vi "Main.vi"() -> ()   [LabVIEW 2023]
doc: "This template is for the Queued Message Handler design pattern.\n\nThe Event Handling Loop generates messages based on user interface actions.\n\nThe Message Handling Loop processes messages generated by the Event Handling Loop, or by other messages. The messages are string values, so new messages can be added easily to the Message Cases case structure in the Message Handling Loop. Each message cluster can also provide an optional value for Message Data, which is a variant that can be converted to whatever message-specific data is required."
uses:
  Drivers/Resideo Gas Valve/Type Definitions/Temperature Control.ctl
  controls/UI Data.ctl
  Drivers/Resideo Gas Valve/Type Definitions/Vesta Info.ctl
  controls/Timer Application Cluster.ctl
  controls/Burner Duty Cycle.ctl
  Hybrid Water Heater/Type Definitions/HEWH MW100 Data Cluster.ctl
  Hybrid Water Heater/Custom Instrument Control/MW100/Type Definitions/HEWH Module 4 Relay Status.ctl
  support/Message Queue/Enqueue Message (Single).vi
  <vilib>/Utility/error.llb/Error Cluster From Error Code.vi
  <vilib>/ErrorRing/Error Ring.xnode
  support/Message Queue/Message Queue.lvlib
  support/User Event - Stop/User Event - Stop.lvlib
panel:
  in  "Disable T2 Control":bool
  in  "Differential Top":dbl=12.0 format="%#_13g"
  in  "Save Rate (ms)":i32=1000
  in  "MW100 Com Port":refnum<visa-resource-name>
  in  "Disable Cycling":bool=TRUE
  in  "Update Vesta Temperature":bool
  in  "VestaTemperature":T1={"Water Heater Temp (°F)"=125, "Differential  (°F)"=25.0} {"Water Heater Temp (°F)" min=32 max=203}
  in  "Burner OFF Time (Seconds)":dbl=60.0
  in  "Burner ON Time (Seconds)":dbl=60.0
  in  "Update Duty Cycle":bool
  out "Data Cluster Output":T2={"Vesta Data Output"={"Temp_W_Raw_U"=0, "Temp_W_Raw_L"=0, "Temperature Water (F)"=0.0, "Temperature Water Compensated (F)"=0.0, "Temperature Ambient (F)"=0.0, "Setpoint Location (F)"=0.0, "Heat Request"="", "Fault Ram"="", "PWM DCDC Value"=0, "Pilot Voltage (mV)"=0.0, "Setpoint Actual (F)"=0.0, "Differential Actual (F)"=0.0, "Setpoint User (F)"=0.0, "Differential User (F)"=0.0, "Termperature FIltered -TCO (F)"=0.0, "Temp_C_Raw_1 - Sensor Voltage"="", "Temp_C_Raw_2 - Sensor Voltage"="", "Chamber Sensor Temperature (F)"=0.0, "LDO Base Temperature (F)"=0.0, "LDO Timer (sec)"=0, "Disabled (0)"=FALSE, "Warming (1)"=FALSE, "Heating (2)"=FALSE, "Cooling Data Write (3)"=FALSE, "Cooling (4)"=FALSE, "Data Read (5)"=FALSE, "N/A"=FALSE, "Temperature Trip (7)"=FALSE, "Burner"=FALSE}, "VestaTemperature"={"Water Heater Temp (°F)"=135, "Differential  (°F)"=10.0}, "Timer Application Data"={"Duty Cycle"={"Burner ON Time (Seconds)"=60.0, "Burner OFF Time (Seconds)"=60.0, "Main Burner Flag"=FALSE, "Burner Power Mode"=0}}, "Data Array"=[], "MW Output"={"TC1-Channel 021"=0.0, "TC2-Channel 022"=0.0, "TC3-Channel 023"=0.0, "TC4-Channel 024"=0.0, "TC5-Channel 025"=0.0, "TC6-Channel 026"=0.0, "TC7-Channel 017"=0.0, "TC8-Channel 028"=0.0, "TC9-Channel 029"=0.0, "TC10-Channel 030"=0.0, "TC Tree Average"=0.0, "TC DWN- Channel 027"=0.0, "RTDin-Channel 031"=0.0, "RTDout-Channel 032"=0.0, "RTDamb-Channel 033"=0.0, "PSI1-Channel 011"=0.0, "PSI2-Channel 012"=0.0, "PSI3-Channel 013"=0.0, "PSI4-Channel 014"=0.0, "UE State-Channel 015"=0.0, "LE State-Channel 016"=0.0, "Module 4 Relay Status Output"={"INTELLIFAUCET TEMP(T)/FLOW(F) (CH 041)"=FALSE, "INTELLIFAUCET READY (CH 042)"=FALSE, "INTELLIFAUCET START (CH 043)"=FALSE, "INTELLIFAUCET STOP (CH 044)"=FALSE, "MAIN POWER RELAY (CH 047)"=FALSE, "NOT USED (CH 045)"=FALSE, "NOT USED (CH 046)"=FALSE, "PURGE VALVE RELAY (CH 048)"=FALSE, "OUTLET VALVE RELAY (CH 049)"=FALSE, "INLET VALVE RELAY (CH 050)"=FALSE, "Intellifaucet (% Open)"=0.0, "Proportioning Valve (%Open)"=0.0, "Intellifaucet Temp Setpoint (F)"=0.0}}} {"VestaTemperature"."Water Heater Temp (°F)" min=32 max=203}
  in  "Vesta Com Port":refnum<visa-resource-name>
  out "Debug":string[](array[string])
  in  "Debug":bool
  in  "Save Data":bool
  in  "Exit":bool
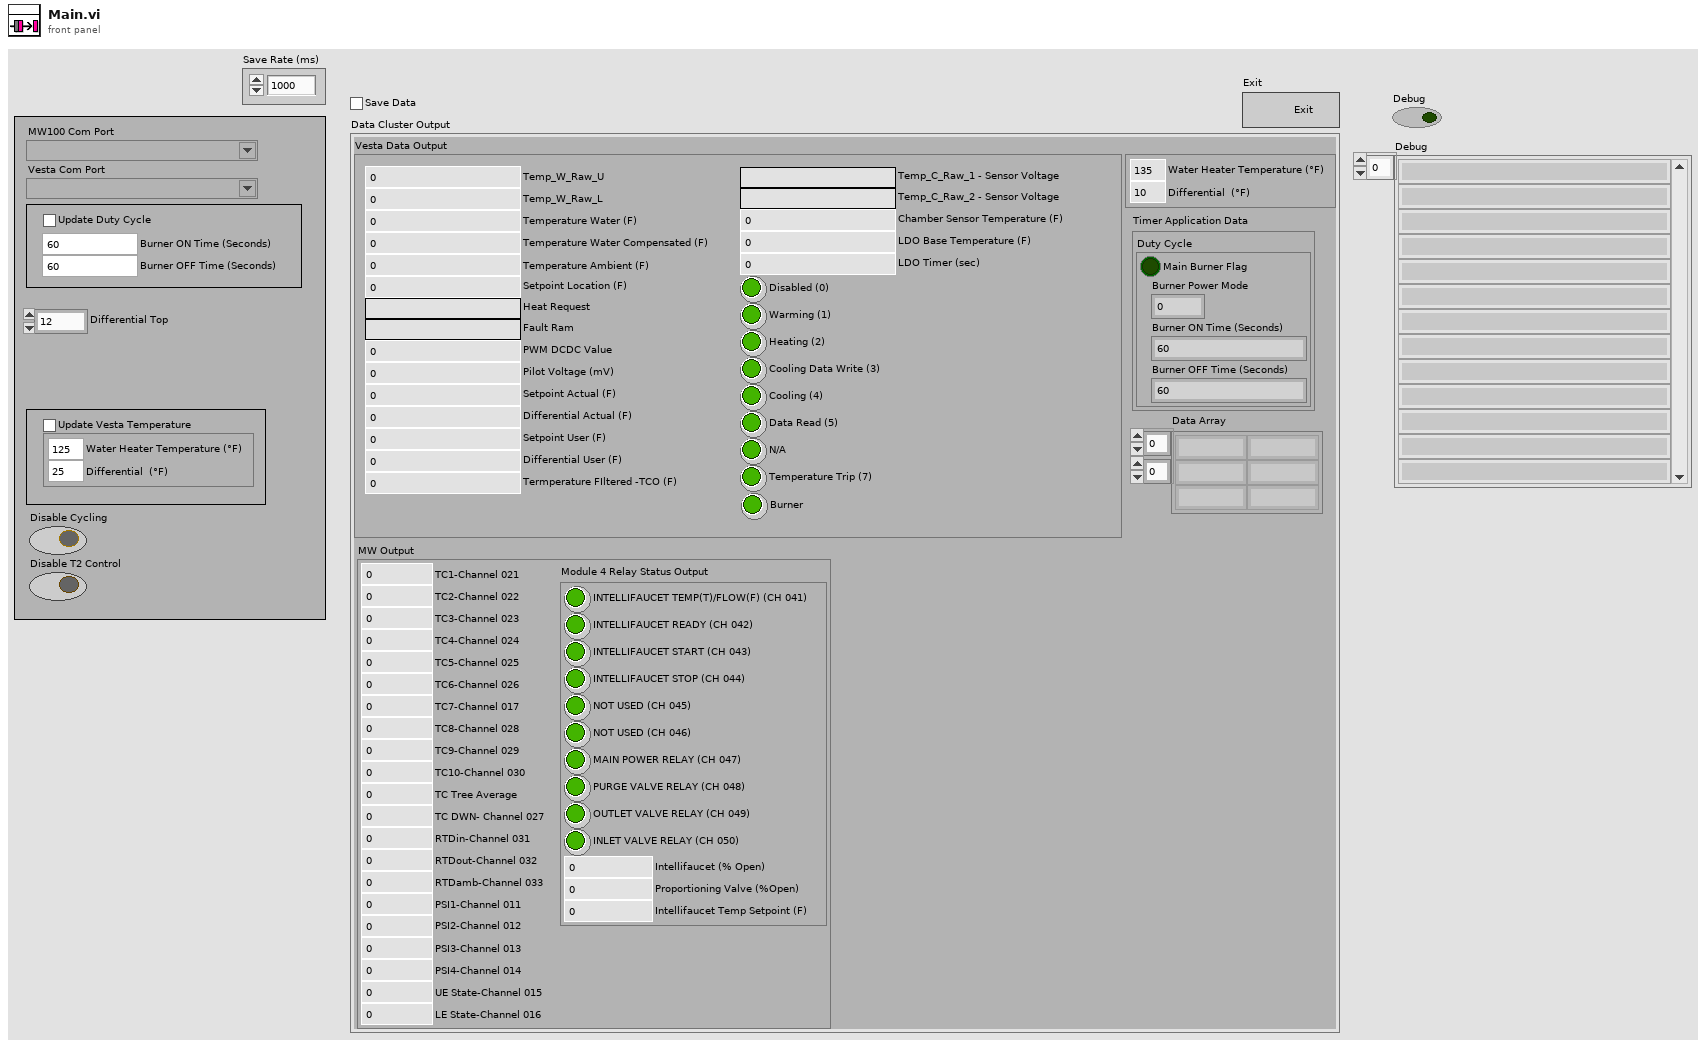
[diagram p1: front panel]
types:
  T1 = typedef "Temperature Control.ctl" = cluster{"Water Heater Temp (°F)":u16, "Differential  (°F)":dbl}
  T2 = typedef "UI Data.ctl" = cluster{"Vesta Data Output":T3, "VestaTemperature":T1, "Timer Application Data":T4, "Data Array":string[][], "MW Output":T6}
  T3 = typedef "Vesta Info.ctl" = cluster{"Temp_W_Raw_U":u16, "Temp_W_Raw_L":u16, "Temperature Water (F)":dbl, "Temperature Water Compensated (F)":dbl, "Temperature Ambient (F)":dbl, "Setpoint Location (F)":dbl, "Heat Request":string, "Fault Ram":string, "PWM DCDC Value":u16, "Pilot Voltage (mV)":dbl, "Setpoint Actual (F)":dbl, "Differential Actual (F)":dbl, "Setpoint User (F)":dbl, "Differential User (F)":dbl, "Termperature FIltered -TCO (F)":dbl, "Temp_C_Raw_1 - Sensor Voltage":string, "Temp_C_Raw_2 - Sensor Voltage":string, "Chamber Sensor Temperature (F)":dbl, "LDO Base Temperature (F)":dbl, "LDO Timer (sec)":i16, "Disabled (0)":bool, "Warming (1)":bool, "Heating (2)":bool, "Cooling Data Write (3)":bool, "Cooling (4)":bool, "Data Read (5)":bool, "N/A":bool, "Temperature Trip (7)":bool, "Burner":bool}
  T4 = typedef "Timer Application Cluster.ctl" = cluster{"Duty Cycle":T5}
  T5 = typedef "Burner Duty Cycle.ctl" = cluster{"Burner ON Time (Seconds)":dbl, "Burner OFF Time (Seconds)":dbl, "Main Burner Flag":bool, "Burner Power Mode":u8}
  T6 = typedef "HEWH MW100 Data Cluster.ctl" = cluster{"TC1-Channel 021":dbl, "TC2-Channel 022":dbl, "TC3-Channel 023":dbl, "TC4-Channel 024":dbl, "TC5-Channel 025":dbl, "TC6-Channel 026":dbl, "TC7-Channel 017":dbl, "TC8-Channel 028":dbl, "TC9-Channel 029":dbl, "TC10-Channel 030":dbl, "TC Tree Average":dbl, "TC DWN- Channel 027":dbl, "RTDin-Channel 031":dbl, "RTDout-Channel 032":dbl, "RTDamb-Channel 033":dbl, "PSI1-Channel 011":dbl, "PSI2-Channel 012":dbl, "PSI3-Channel 013":dbl, "PSI4-Channel 014":dbl, "UE State-Channel 015":dbl, "LE State-Channel 016":dbl, "Module 4 Relay Status Output":T7}
  T7 = typedef "HEWH Module 4 Relay Status.ctl" = cluster{"INTELLIFAUCET TEMP(T)/FLOW(F) (CH 041)":bool, "INTELLIFAUCET READY (CH 042)":bool, "INTELLIFAUCET START (CH 043)":bool, "INTELLIFAUCET STOP (CH 044)":bool, "MAIN POWER RELAY (CH 047)":bool, "NOT USED (CH 045)":bool, "NOT USED (CH 046)":bool, "PURGE VALVE RELAY (CH 048)":bool, "OUTLET VALVE RELAY (CH 049)":bool, "INLET VALVE RELAY (CH 050)":bool, "Intellifaucet (% Open)":dbl, "Proportioning Valve (%Open)":dbl, "Intellifaucet Temp Setpoint (F)":dbl}
  T8 = typedef "Message Queue.lvlib/All Message Queues.ctl" = cluster{"UI":refnum<queue>, "DataSave":refnum<queue>, "Vesta":refnum<queue>, "MW100":refnum<queue>}
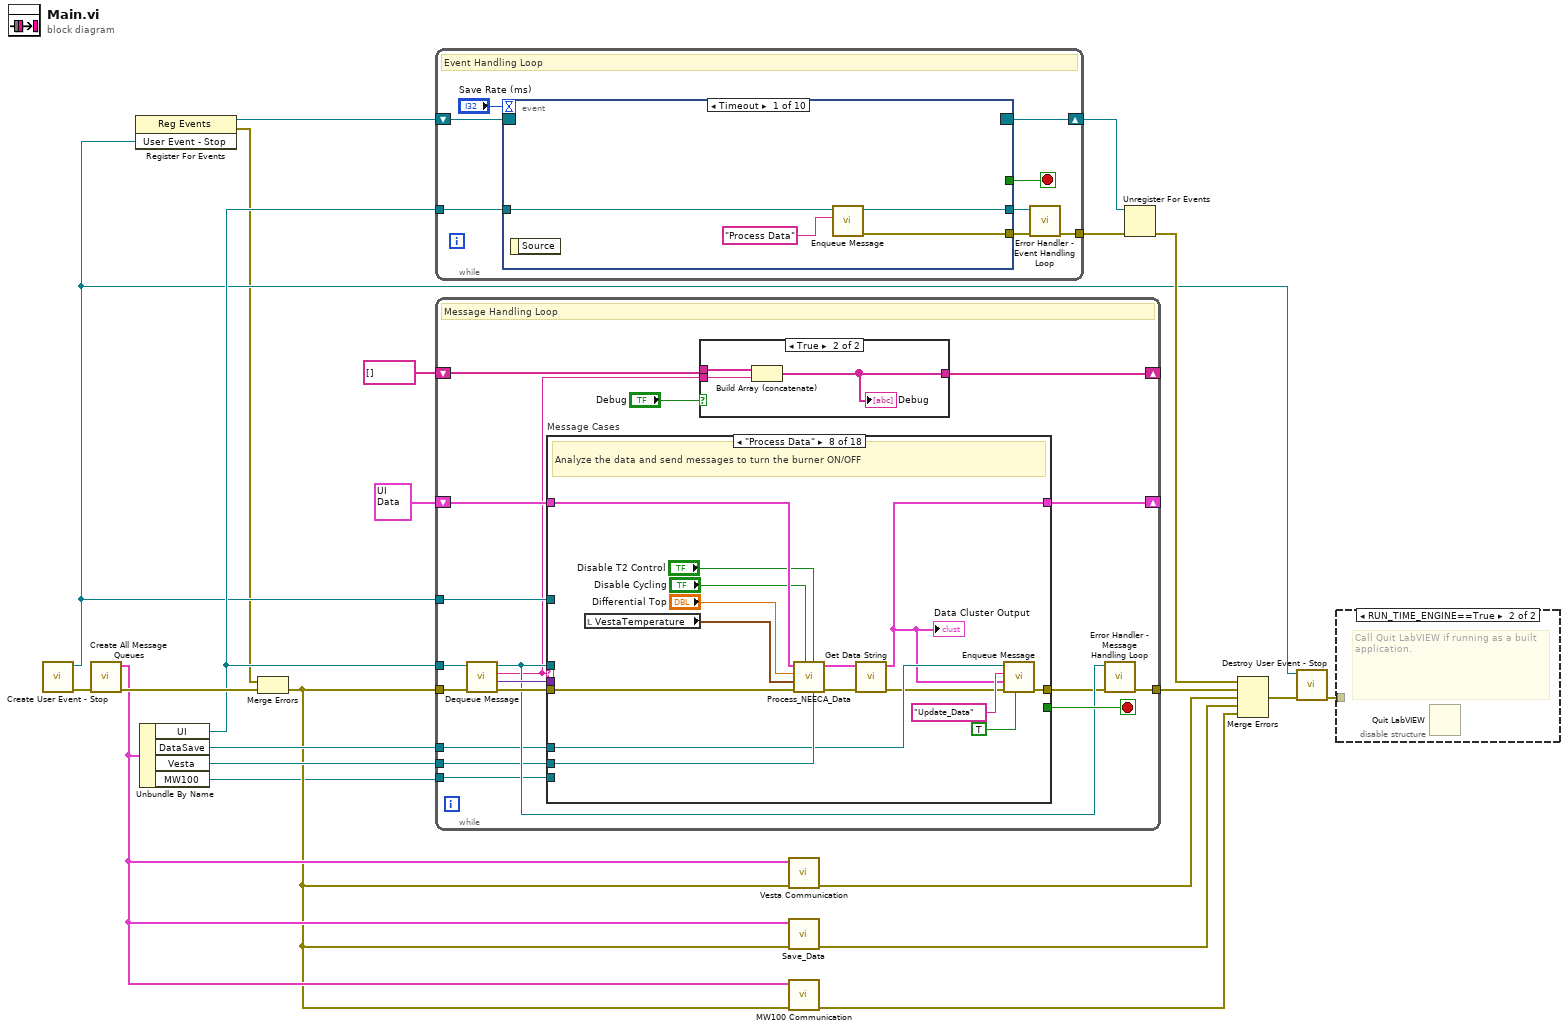
[diagram p0: block diagram]
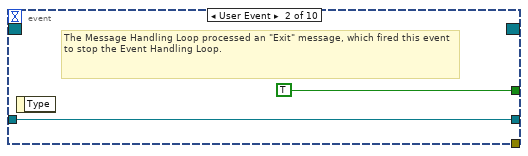
[diagram p3: hidden frame]
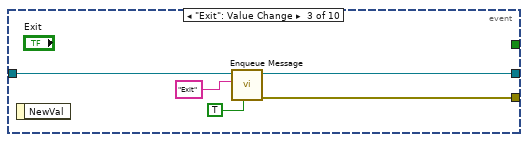
[diagram p4: hidden frame]
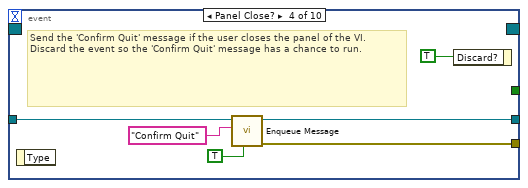
[diagram p5: hidden frame]
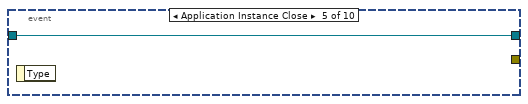
[diagram p6: hidden frame]
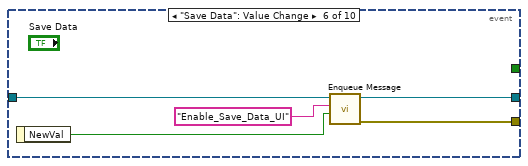
[diagram p7: hidden frame]
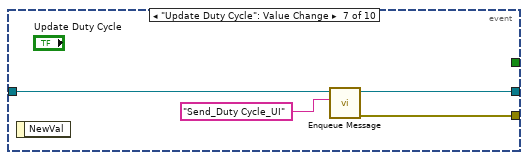
[diagram p8: hidden frame]
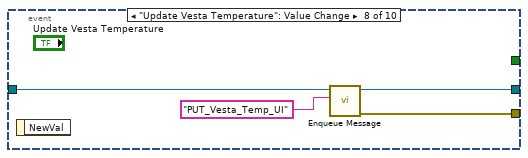
[diagram p9: hidden frame]
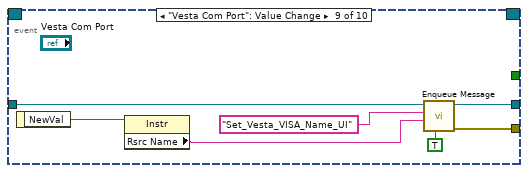
[diagram p10: hidden frame]
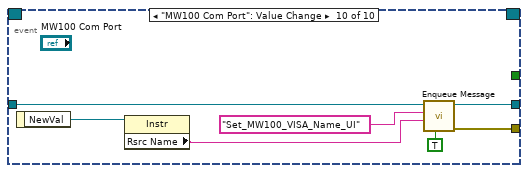
[diagram p11: hidden frame]
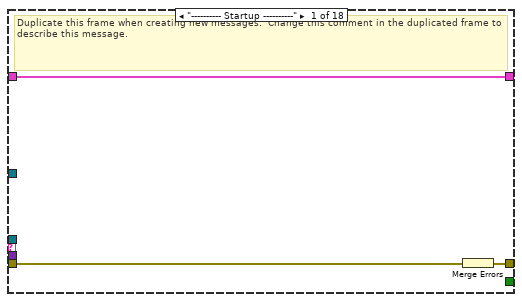
[diagram p13: hidden frame]
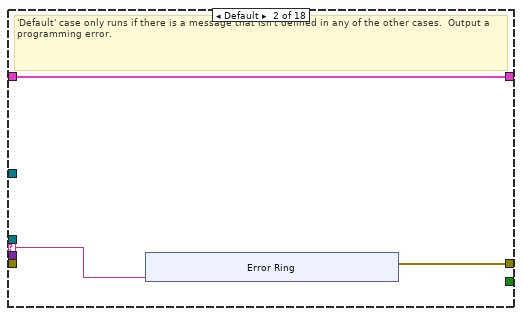
[diagram p14: hidden frame]
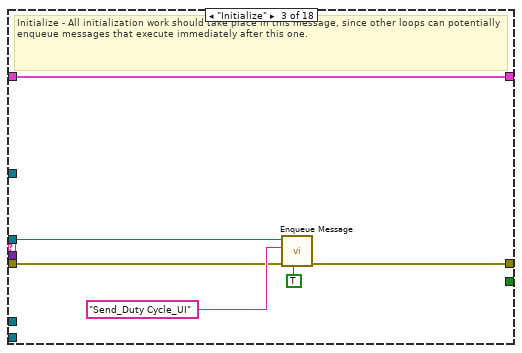
[diagram p15: hidden frame]
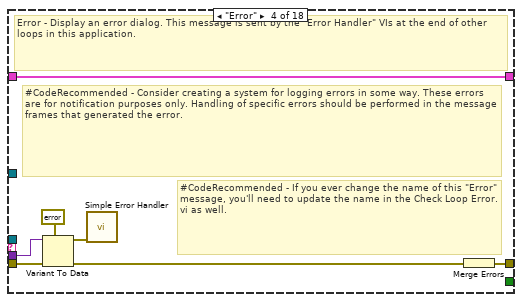
[diagram p16: hidden frame]
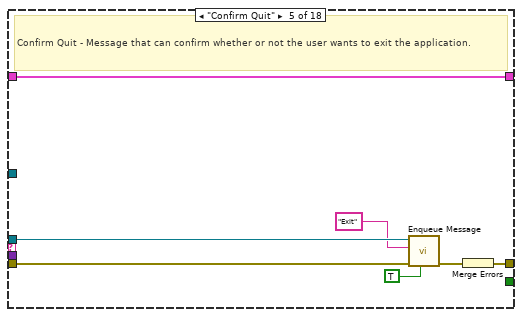
[diagram p17: hidden frame]
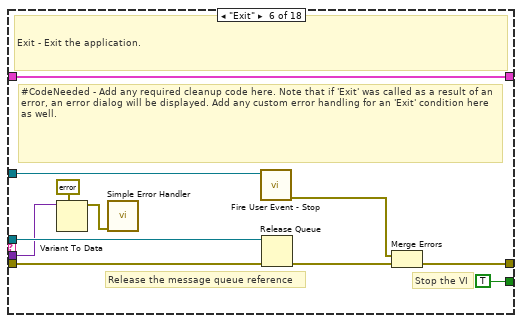
[diagram p18: hidden frame]
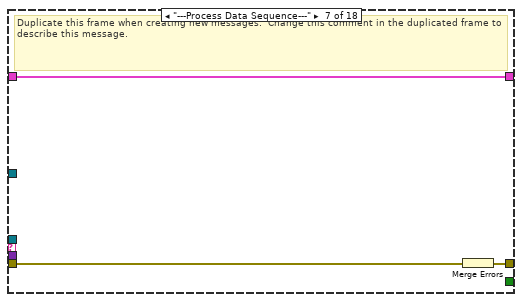
[diagram p19: hidden frame]
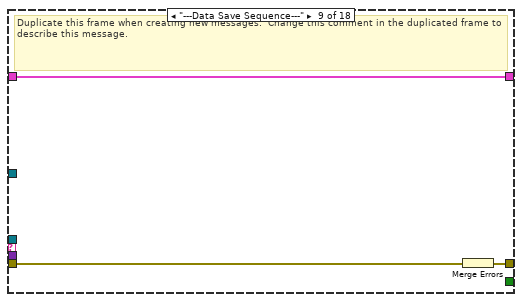
[diagram p20: hidden frame]
diagram:
  n1 = call "Create User Event - Stop.vi"() -> ("error out"=w19:errorcluster, "User Event - Stop"=w11:refnum<user-event>)  [unwired: 10 in]
  n2 = call "Create All Message Queues.vi"("error in (no error)"=w19) -> ("error out"=w22:errorcluster, "Message Queues out"=w4:T8)  [unwired: 9 in]
  n3 = register-events(w11) -> (reference out=w12:refnum<event-registration>, error out=w10:errorcluster)  [unwired: 2 in]
  n4 = Unbundle By Name(w4) -> ("UI"=w20:refnum<queue>, "DataSave"=w9:refnum<queue>, "Vesta"=w6:refnum<queue>, "MW100"=w1:refnum<queue>)
  n5 = Merge Errors(w10, w22) -> (w3:errorcluster)
  n6 = while {
    tunnel: w20 -> [w30]
    shift-right: [w28] -> w16
    shift-left: w12 -> [w29]
    tunnel: [w24] -> w13
    stop <- w26 stop-if-true
    # "Event Handling Loop"
    n7 = event shown="[0] Timeout" {
      selector: w29 -> [_ _ _ _ _ _ _ _ _ _]
      dyn-events: [_ _ _ _ _ _ _ _ _ _] -> w28
      timeout: "Save Rate (ms)" -> [_ _ _ _ _ _ _ _ _ _]
      tunnel: [_ TRUE ("Discard?") _ _ _ _ _ _ _ _] -> w26
      tunnel: w30 -> [w33 w36 w41 w46 w48 w53 w57 w61 w68 w75]
      tunnel: [w31 _ w40 w45 _ w50 w54 w58 w65 w72] -> w27
      tunnel: [w32 w36 w39 w44 w48 w52 w56 w60 w67 w74] -> w25
      event Timeout {
        n8 = event-data() -> ()  [unwired: 1 in, 1 out]
        n9 = call-poly "Enqueue Message.vi"("Message"="Process Data", "Message Queue"=w33) -> ("error out"=w31:errorcluster, "dup Message Queue"=w32:refnum<queue>)  [unwired: 8 in]
      }
      event User Event {
        # "The Message Handling Loop processed an \"Exit\" message, which fired this event to stop the Event Handling Loop."
        n10 = event-data() -> ()  [unwired: 1 in, 1 out]
      }
      event "Exit": Value Change {
        n11 = event-data() -> ()  [unwired: 1 in, 1 out]
        n12 = call-poly "Enqueue Message.vi"("Priority Message? (F)"=TRUE, "Message"="Exit", "Message Queue"=w41) -> ("error out"=w40:errorcluster, "dup Message Queue"=w39:refnum<queue>)  [unwired: 7 in]
      }
      event Panel Close? {
        # "Send the 'Confirm Quit' message if the user closes the panel of the VI. Discard the event so the 'Confirm Quit' message has a chance to run."
        n13 = event-data() -> ()  [unwired: 1 in, 1 out]
        n14 = call-poly "Enqueue Message.vi"("Priority Message? (F)"=TRUE, "Message"="Confirm Quit", "Message Queue"=w46) -> ("error out"=w45:errorcluster, "dup Message Queue"=w44:refnum<queue>)  [unwired: 7 in]
        n15 = event-data("Discard?"=TRUE) -> ()  [unwired: 1 in, 1 out]
      }
      event Application Instance Close {
        n16 = event-data() -> ()  [unwired: 1 in, 1 out]
      }
      event "Save Data": Value Change {
        n17 = event-data() -> ("NewVal"=w49:bool)  [unwired: 1 in]
        n18 = call-poly "Enqueue Message.vi"("Message Data"=w49, "Message"="Enable_Save_Data_UI", "Message Queue"=w53) -> ("error out"=w50:errorcluster, "dup Message Queue"=w52:refnum<queue>)  [unwired: 7 in]
      }
      event "Update Duty Cycle": Value Change {
        n19 = event-data() -> ()  [unwired: 1 in, 1 out]
        n20 = call-poly "Enqueue Message.vi"("Message"="Send_Duty Cycle_UI", "Message Queue"=w57) -> ("error out"=w54:errorcluster, "dup Message Queue"=w56:refnum<queue>)  [unwired: 8 in]
      }
      event "Update Vesta Temperature": Value Change {
        n21 = event-data() -> ()  [unwired: 1 in, 1 out]
        n22 = call-poly "Enqueue Message.vi"("Message"="PUT_Vesta_Temp_UI", "Message Queue"=w61) -> ("error out"=w58:errorcluster, "dup Message Queue"=w60:refnum<queue>)  [unwired: 8 in]
      }
      event "Vesta Com Port": Value Change {
        n23 = event-data() -> ("NewVal"=w64:refnum<visa-resource-name>)  [unwired: 1 in]
        n24 = property class="Instr"(reference=w64) -> ("Rsrc Name"=w63:string)  [unwired: 1 in, 2 out]
        n25 = call-poly "Enqueue Message.vi"("Priority Message? (F)"=TRUE, "Message Data"=w63, "Message"="Set_Vesta_VISA_Name_UI", "Message Queue"=w68) -> ("error out"=w65:errorcluster, "dup Message Queue"=w67:refnum<queue>)  [unwired: 6 in]
      }
      event "MW100 Com Port": Value Change {
        n26 = event-data() -> ("NewVal"=w71:refnum<visa-resource-name>)  [unwired: 1 in]
        n27 = property class="Instr"(reference=w71) -> ("Rsrc Name"=w69:string)  [unwired: 1 in, 2 out]
        n28 = call-poly "Enqueue Message.vi"("Priority Message? (F)"=TRUE, "Message Data"=w69, "Message"="Set_MW100_VISA_Name_UI", "Message Queue"=w75) -> ("error out"=w72:errorcluster, "dup Message Queue"=w74:refnum<queue>)  [unwired: 6 in]
      }
    }
    n29 = call "Error Handler - Event Handling Loop.vi"("error in (no error)"=w27, "Message Queue"=w25) -> ("dup error in"=w24:errorcluster)  [unwired: 8 in, 1 out]
  }
  n30 = while {
    tunnel: w20 -> [w86]
    shift-right: [w92] -> _
    shift-left: T2 {"Vesta Data Output"={"Temp_W_Raw_U"=0, "Temp_W_Raw_L"=0, "Temperature Water (F)"=0.0, "Temperature Water Compensated (F)"=0.0, "Temperature Ambient (F)"=0.0, "Setpoint Location (F)"=0.0, "Heat Request"="", "Fault Ram"="", "PWM DCDC Value"=0, "Pilot Voltage (mV)"=0.0, "Setpoint Actual (F)"=0.0, "Differential Actual (F)"=0.0, "Setpoint User (F)"=0.0, "Differential User (F)"=0.0, "Termperature FIltered -TCO (F)"=0.0, "Temp_C_Raw_1 - Sensor Voltage"="", "Temp_C_Raw_2 - Sensor Voltage"="", "Chamber Sensor Temperature (F)"=0.0, "LDO Base Temperature (F)"=0.0, "LDO Timer (sec)"=0, "Disabled (0)"=FALSE, "Warming (1)"=FALSE, "Heating (2)"=FALSE, "Cooling Data Write (3)"=FALSE, "Cooling (4)"=FALSE, "Data Read (5)"=FALSE, "N/A"=FALSE, "Temperature Trip (7)"=FALSE, "Burner"=FALSE}, "VestaTemperature"={"Water Heater Temp (°F)"=135, "Differential  (°F)"=10.0}, "Timer Application Data"={"Duty Cycle"={"Burner ON Time (Seconds)"=60.0, "Burner OFF Time (Seconds)"=60.0, "Main Burner Flag"=FALSE, "Burner Power Mode"=0}}, "Data Array"=[], "MW Output"={"TC1-Channel 021"=0.0, "TC2-Channel 022"=0.0, "TC3-Channel 023"=0.0, "TC4-Channel 024"=0.0, "TC5-Channel 025"=0.0, "TC6-Channel 026"=0.0, "TC7-Channel 017"=0.0, "TC8-Channel 028"=0.0, "TC9-Channel 029"=0.0, "TC10-Channel 030"=0.0, "TC Tree Average"=0.0, "TC DWN- Channel 027"=0.0, "RTDin-Channel 031"=0.0, "RTDout-Channel 032"=0.0, "RTDamb-Channel 033"=0.0, "PSI1-Channel 011"=0.0, "PSI2-Channel 012"=0.0, "PSI3-Channel 013"=0.0, "PSI4-Channel 014"=0.0, "UE State-Channel 015"=0.0, "LE State-Channel 016"=0.0, "Module 4 Relay Status Output"={"INTELLIFAUCET TEMP(T)/FLOW(F) (CH 041)"=FALSE, "INTELLIFAUCET READY (CH 042)"=FALSE, "INTELLIFAUCET START (CH 043)"=FALSE, "INTELLIFAUCET STOP (CH 044)"=FALSE, "MAIN POWER RELAY (CH 047)"=FALSE, "NOT USED (CH 045)"=FALSE, "NOT USED (CH 046)"=FALSE, "PURGE VALVE RELAY (CH 048)"=FALSE, "OUTLET VALVE RELAY (CH 049)"=FALSE, "INLET VALVE RELAY (CH 050)"=FALSE, "Intellifaucet (% Open)"=0.0, "Proportioning Valve (%Open)"=0.0, "Intellifaucet Temp Setpoint (F)"=0.0}}} ("Data Cluster") -> [w93]
    tunnel: w11 -> [w90]
    tunnel: w3 -> [w89]
    tunnel: [w84] -> w21
    tunnel: w9 -> [w82]
    shift-right: [w78] -> _
    shift-left: string[] [] -> [w80]
    tunnel: w6 -> [w77]
    tunnel: w1 -> [w76]
    stop <- w91 stop-if-true
    # "Message Handling Loop"
    n31 = call "Dequeue Message.vi"("error in (no error)"=w89, "Message Queue"=w86) -> ("error out"=w88:errorcluster, "Message Data"=w87:variant, "Message"=w79:string, "dup Message Queue"=w85:refnum<queue>)  [unwired: 6 in]
    n32 = case "Message Cases" shown="\"Process Data\"" w79 {
      selector: w79 -> [_ w101 _ _ _ _ _ _ _ _ _ _ _ _ _ _ _ _]
      tunnel: w85 -> [_ _ w112 _ w126 w141 _ _ _ _ _ _ _ _ _ _ _ _]
      tunnel: w88 -> [w100 _ w114 w123 w130 w134 w144 w158 w162 w167 w176 w180 w196 w202 w210 w213 w218 w231]
      tunnel: [w98 w102 w113 w117 w128 w137 w142 w154 w160 w172 w174 w186 w197 w203 w204 w211 w223 w225] -> w83
      tunnel: w93 -> [w99 w103 w116 w122 w129 w140 w143 w157 w161 w173 w175 w187 w191 w201 w207 w212 w224 w230]
      tunnel: [w99 w103 w116 w122 w129 w140 w143 w149 w161 w173 w175 w187 w190 w200 w206 w212 w224 w229] -> w92
      tunnel: [_ _ _ _ _ TRUE _ _ _ _ _ _ _ _ _ _ _ _] -> w91
      tunnel: w87 -> [_ _ _ w121 _ w131 _ _ _ w164 _ w178 _ _ w209 _ w216 w228]
      tunnel: w90 -> [_ _ _ _ _ w136 _ _ _ _ _ _ _ _ _ _ _ _]
      tunnel: w82 -> [_ _ _ _ _ _ _ w153 _ w169 _ _ _ _ _ _ _ _]
      tunnel: w77 -> [_ _ _ _ _ _ _ w159 _ _ _ w182 w192 _ _ _ _ _]
      tunnel: w76 -> [_ _ _ _ _ _ _ _ _ _ _ _ _ _ _ _ w215 _]
      frame "---------- Startup ----------" {
        # "Duplicate this frame when creating new messages.  Change this comment in the duplicated frame to describe this message."
        n33 = Merge Errors(w100) -> (w98:errorcluster)
      }
      frame Default {
        # "'Default' case only runs if there is a message that isn't defined in any of the other cases.  Output a programming error."
        n34 = xnode "Error Ring"("parameter 0"=w101) -> ("error out"=w102:errorcluster)
      }
      frame "Initialize" {
        # "Initialize - All initialization work should take place in this message, since other loops can potentially enqueue messages that execute immediately after this one."
        n35 = call-poly "Enqueue Message.vi"("Priority Message? (F)"=TRUE, "error in (no error)"=w114, "Message"="Send_Duty Cycle_UI", "Message Queue"=w112) -> ("error out"=w113:errorcluster)  [unwired: 6 in, 1 out]
      }
      frame "Error" {
        # "#CodeRecommended - If you ever change the name of this \"Error\" message, you'll need to update the name in the Check Loop Error.vi as well."
        # "#CodeRecommended - Consider creating a system for logging errors in some way. These errors are for notification purposes only. Handling of specific errors should be performed in the message frames that generated the error."
        # "Error - Display an error dialog. This message is sent by the \"Error Handler\" VIs at the end of other loops in this application."
        n36 = Variant To Data(error in=w123, type=errorcluster {"status"=FALSE, "code"=0, "source"=""} ("error constant"), Variant=w121) -> (data=w119:errorcluster, error out=w118:errorcluster)
        n37 = call <vilib>:"Simple Error Handler.vi"("error in (no error)"=w119) -> ()  [unwired: 4 in, 5 out]
        n38 = Merge Errors(w118) -> (w117:errorcluster)
      }
      frame "Confirm Quit" {
        # "Confirm Quit - Message that can confirm whether or not the user wants to exit the application."
        n39 = call-poly "Enqueue Message.vi"("Priority Message? (F)"=TRUE, "error in (no error)"=w130, "Message"="Exit", "Message Queue"=w126) -> ("error out"=w127:errorcluster)  [unwired: 6 in, 1 out]
        n40 = Merge Errors(w127) -> (w128:errorcluster)
      }
      frame "Exit" {
        # "Stop the VI"
        # "Release the message queue reference"
        # "#CodeNeeded - Add any required cleanup code here. Note that if 'Exit' was called as a result of an error, an error dialog will be displayed. Add any custom error handling for an 'Exit' condition here as well."
        # "Exit - Exit the application."
        n41 = Variant To Data(type=errorcluster {"status"=FALSE, "code"=0, "source"=""} ("error constant"), Variant=w131) -> (data=w132:errorcluster)  [unwired: 1 in, 1 out]
        n42 = call <vilib>:"Simple Error Handler.vi"("error in (no error)"=w132) -> ()  [unwired: 4 in, 5 out]
        n43 = call "Fire User Event - Stop.vi"("User Event - Stop"=w136) -> ("error out"=w135:errorcluster)  [unwired: 10 in]
        n44 = Release Queue(queue=w141, error in (no error)=w134) -> (error out=w138:errorcluster)  [unwired: 1 in, 2 out]
        n45 = Merge Errors(w135, w138) -> (w137:errorcluster)
      }
      frame "---Process Data Sequence---" {
        # "Duplicate this frame when creating new messages.  Change this comment in the duplicated frame to describe this message."
        n46 = Merge Errors(w144) -> (w142:errorcluster)
      }
      frame "Process Data" {
        # "Analyze the data and send messages to turn the burner ON/OFF"
        n47 = local read "VestaTemperature"() -> (w145:T1)
        n48 = call "Process_NEECA_Data.vi"("Vesta in"=w159, "Disable T2 Control"="Disable T2 Control", "Disable Cycling"="Disable Cycling", "error in (no error)"=w158, "VestaTemperature Fixed"=w145, "Differential_Top"="Differential Top", "Data Cluster"=w157) -> ("error out"=w152:errorcluster, "Data Cluster Output"=w150:T2)  [unwired: 3 in]
        n49 = call "Get Data String.vi"("error in (no error)"=w152, "Data Cluster Out"=w150) -> ("error out"=w151:errorcluster, "Data Cluster Output"=w149:T2)  [unwired: 8 in]
        "Data Cluster Output" <- w149
        n50 = call-poly "Enqueue Message.vi"("Priority Message? (F)"=TRUE, "error in (no error)"=w151, "Message Data"=w149, "Message"="Update_Data", "Message Queue"=w153) -> ("error out"=w154:errorcluster)  [unwired: 5 in, 1 out]
      }
      frame "---Data Save Sequence---" {
        # "Duplicate this frame when creating new messages.  Change this comment in the duplicated frame to describe this message."
        n51 = Merge Errors(w162) -> (w160:errorcluster)
      }
      frame "Enable_Save_Data_UI" {
        # "Reset the Timer"
        n52 = Variant To Data(error in=w167, type=FALSE, Variant=w164) -> (data=w163:bool, error out=w166:errorcluster)
        n53 = call-poly "Enqueue Message.vi"("Priority Message? (F)"=TRUE, "error in (no error)"=w166, "Message Data"=w163, "Message"="Enable_Save_Data", "Message Queue"=w169) -> ("error out"=w171:errorcluster)  [unwired: 5 in, 1 out]
        n54 = Merge Errors(w171) -> (w172:errorcluster)
      }
      frame "---Vesta Sequence---" {
        # "Duplicate this frame when creating new messages.  Change this comment in the duplicated frame to describe this message."
        n55 = Merge Errors(w176) -> (w174:errorcluster)
      }
      frame "Set_Vesta_VISA_Name_UI" {
        # "Something Else - Replace this message with functionality for your own application."
        n56 = Variant To Data(error in=w180, type="", Variant=w178) -> (data=w177:string, error out=w179:errorcluster)
        n57 = call-poly "Enqueue Message.vi"("Priority Message? (F)"=TRUE, "error in (no error)"=w179, "Message Data"=w177, "Message"="Set_Vesta_VISA_Name", "Message Queue"=w182) -> ("error out"=w185:errorcluster)  [unwired: 5 in, 1 out]
        n58 = Merge Errors(w185) -> (w186:errorcluster)
      }
      frame "PUT_Vesta_Temp_UI" {
        # "Something Else - Replace this message with functionality for your own application."
        n59 = Unbundle By Name("VestaTemperature") -> ("Differential  (°F)"=w188:dbl)
        n60 = Bundle By Name(cluster=w191, "VestaTemperature.Differential  (°F)"=w188) -> (w190:T2)
        n61 = call-poly "Enqueue Message.vi"("Priority Message? (F)"=TRUE, "error in (no error)"=w196, "Message Data"="VestaTemperature", "Message"="PUT_Vesta_Temp", "Message Queue"=w192) -> ("error out"=w195:errorcluster)  [unwired: 5 in, 1 out]
        n62 = Merge Errors(w195) -> (w197:errorcluster)
      }
      frame "Send_Duty Cycle_UI" {
        # "Something Else - Replace this message with functionality for your own application."
        n63 = Bundle By Name(cluster=w201, "Timer Application Data.Duty Cycle.Burner ON Time (Seconds)"="Burner ON Time (Seconds)", "Timer Application Data.Duty Cycle.Burner OFF Time (Seconds)"="Burner OFF Time (Seconds)") -> (w200:T2)
        n64 = Merge Errors(w202) -> (w203:errorcluster)
      }
      frame "DisplayValuesFromVesta" {
        n65 = Variant To Data(error in=w210, type=T3 {"Temp_W_Raw_U"=0, "Temp_W_Raw_L"=0, "Temperature Water (F)"=0.0, "Temperature Water Compensated (F)"=0.0, "Temperature Ambient (F)"=0.0, "Setpoint Location (F)"=0.0, "Heat Request"="", "Fault Ram"="", "PWM DCDC Value"=0, "Pilot Voltage (mV)"=0.0, "Setpoint Actual (F)"=0.0, "Differential Actual (F)"=0.0, "Setpoint User (F)"=0.0, "Differential User (F)"=0.0, "Termperature FIltered -TCO (F)"=0.0, "Temp_C_Raw_1 - Sensor Voltage"="", "Temp_C_Raw_2 - Sensor Voltage"="", "Chamber Sensor Temperature (F)"=0.0, "LDO Base Temperature (F)"=0.0, "LDO Timer (sec)"=0, "Disabled (0)"=FALSE, "Warming (1)"=FALSE, "Heating (2)"=FALSE, "Cooling Data Write (3)"=FALSE, "Cooling (4)"=FALSE, "Data Read (5)"=FALSE, "N/A"=FALSE, "Temperature Trip (7)"=FALSE, "Burner"=FALSE} ("Vesta Data Output"), Variant=w209) -> (data=w205:T3, error out=w204:errorcluster)
        n66 = Bundle By Name(cluster=w207, "Vesta Data Output"=w205) -> (w206:T2)
      }
      frame "---MW100 Sequence---" {
        # "Duplicate this frame when creating new messages.  Change this comment in the duplicated frame to describe this message."
        n67 = Merge Errors(w213) -> (w211:errorcluster)
      }
      frame "Set_MW100_VISA_Name_UI" {
        # "Something Else - Replace this message with functionality for your own application."
        n68 = Variant To Data(error in=w218, type="", Variant=w216) -> (data=w214:string, error out=w217:errorcluster)
        n69 = call-poly "Enqueue Message.vi"("Priority Message? (F)"=TRUE, "error in (no error)"=w217, "Message Data"=w214, "Message"="Set_MW100_VISA_Name", "Message Queue"=w215) -> ("error out"=w222:errorcluster)  [unwired: 5 in, 1 out]
        n70 = Merge Errors(w222) -> (w223:errorcluster)
      }
      frame "DisplayValuesFromMW100" {
        # "Duplicate this frame when creating new messages.  Change this comment in the duplicated frame to describe this message."
        n71 = Variant To Data(error in=w231, type=T6 {"TC1-Channel 021"=0.0, "TC2-Channel 022"=0.0, "TC3-Channel 023"=0.0, "TC4-Channel 024"=0.0, "TC5-Channel 025"=0.0, "TC6-Channel 026"=0.0, "TC7-Channel 017"=0.0, "TC8-Channel 028"=0.0, "TC9-Channel 029"=0.0, "TC10-Channel 030"=0.0, "TC Tree Average"=0.0, "TC DWN- Channel 027"=0.0, "RTDin-Channel 031"=0.0, "RTDout-Channel 032"=0.0, "RTDamb-Channel 033"=0.0, "PSI1-Channel 011"=0.0, "PSI2-Channel 012"=0.0, "PSI3-Channel 013"=0.0, "PSI4-Channel 014"=0.0, "UE State-Channel 015"=0.0, "LE State-Channel 016"=0.0, "Module 4 Relay Status Output"={"INTELLIFAUCET TEMP(T)/FLOW(F) (CH 041)"=FALSE, "INTELLIFAUCET READY (CH 042)"=FALSE, "INTELLIFAUCET START (CH 043)"=FALSE, "INTELLIFAUCET STOP (CH 044)"=FALSE, "MAIN POWER RELAY (CH 047)"=FALSE, "NOT USED (CH 045)"=FALSE, "NOT USED (CH 046)"=FALSE, "PURGE VALVE RELAY (CH 048)"=FALSE, "OUTLET VALVE RELAY (CH 049)"=FALSE, "INLET VALVE RELAY (CH 050)"=FALSE, "Intellifaucet (% Open)"=0.0, "Proportioning Valve (%Open)"=0.0, "Intellifaucet Temp Setpoint (F)"=0.0}} ("MW Output"), Variant=w228) -> (data=w226:T6, error out=w225:errorcluster)
        n72 = Bundle By Name(cluster=w230, "MW Output"=w226) -> (w229:T2)
      }
    }
    n73 = case shown="True" "Debug" {
      tunnel: w79 -> [_ w97]
      tunnel: w80 -> [w94 w96]
      tunnel: [w94 w95] -> w78
      frame False {
      }
      frame True {
        n74 = Build Array (concatenate)(w96, w97) -> (w95:string[])
        "Debug" <- w95
      }
    }
    n75 = call "Error Handler - Message Handling Loop.vi"("error in (no error)"=w83, "Message Queue"=w85) -> ("dup error in"=w84:errorcluster)  [unwired: 8 in, 1 out]
  }
  n76 = call "Vesta Communication.vi"("error in (no error)"=w3, "Message Queues out"=w4) -> ("error out"=w7:errorcluster)  [unwired: 9 in]
  n77 = call "Save_Data.vi"("error in (no error)"=w3, "Message Queues out"=w4) -> ("error out"=w5:errorcluster)  [unwired: 9 in]
  n78 = call "MW100 Communication.vi"("error in (no error)"=w3, "Message Queues out"=w4) -> ("error out"=w2:errorcluster)  [unwired: 9 in]
  n79 = Unregister For Events(event registration refnum=w16, error in=w13) -> (error out=w17:errorcluster)
  n80 = Merge Errors(w17, w21, w7, w5, w2) -> (w18:errorcluster)
  n81 = call "Destroy User Event - Stop.vi"("error in (no error)"=w18, "User Event - Stop"=w11) -> ("error out"=w14:errorcluster)  [unwired: 9 in]
  n82 = disable-structure shown="RUN_TIME_ENGINE==True" {
    disable-tunnel: w14 -> [_ _]
    frame condition #0 (active) {
    }
    frame condition #1 {
      # "Call Quit LabVIEW if running as a built application."
      n83 = Quit LabVIEW() -> ()  [unwired: 1 in]
    }
  }
